vi "Perform Action.vi"(8 "error in":errorcluster, 10 "Input":variant, 11 "AI Voltage DAQmx Cont CFG Simulated in":refnum<class "AI Voltage DAQmx Cont CFG Simulated.lvclass">) -> (0 "error out":errorcluster, 2 "Output":variant, 3 "AI Voltage DAQmx Cont CFG Simulated out":refnum<class "AI Voltage DAQmx Cont CFG Simulated.lvclass">)   [LabVIEW 2023, in "DAQmx Simulated CFGs.lvlib" / "AI Voltage DAQmx Cont CFG Simulated.lvclass"]
uses:
  DAQmx/DAQmx BufferLastReadsDBL/DAQmx BufferLastReadsDBL.lvclass/DAQmx BufferLastReadsDBL.ctl
  DAQmx/DAQmx Base CFG/DAQmx Base CFG.lvclass/DAQmx Base CFG.ctl
  Configuration/Configuration Semaphore/CFG Semaphore.lvclass/CFG Semaphore.ctl
  <vilib>/JDP Science/JSONtext/Find Item.vi
  <vilib>/JDP Science/JSONtext/Next JSON Value.vi
  <vilib>/JDP Science/JSONtext/String Subset.vi
  <vilib>/JDP Science/JSONtext/Parsing/Advance past next JSON Value (inlined COPY).vi
  <vilib>/JDP Science/JSONtext/Parsing/Advance past whitespace.vi
  <vilib>/JDP Science/JSONtext/Parsing/Advance past String.vi
  <vilib>/JDP Science/JSONtext/Parsing/Advance past Number.vi
  <vilib>/JDP Science/JSONtext/Parsing/Advance past Line Ending.vi
  <vilib>/JDP Science/JSONtext/Parsing/Parse Full Path or Item Name.vi
  <vilib>/JDP Science/JSONtext/Parsing/Advance past Array.vi
  <vilib>/JDP Science/JSONtext/Parsing/Advance past Object.vi
  <vilib>/JDP Science/JSONtext/support/Error Cluster From Code.vi
  <vilib>/JDP Science/JSONtext/Offset/Find Item Locations by Path.vi
  <vilib>/JDP Science/JSONtext/JSON text to Variant.vi
  <vilib>/DAQmx/miscellaneous.llb/DAQmx Fill In Error Info.vi
  <vilib>/JDP Science/JSONtext/LVClass Serializer/JSONtext LVClass Serializer.lvclass
  AI Voltage DAQmx Cont CFG Simulated.lvclass
  AI Voltage DAQmx Cont CFG Simulated.lvclass/AI Voltage DAQmx Cont CFG Simulated.ctl
  45e9973d-d2d9-4ea1-97eb-1b57adbb2603.vi
  DAQmx/DAQmx BufferLastReadsDBL/DAQmx BufferLastReadsDBL.lvclass
  DAQmx/BufferLastReadingsDBL/BufferLastReadsDBL.lvclass
  Configuration/Configuration JSON/Configuration JSON Base/CFG JSON.lvclass
  0cc4d47a-a0da-4a28-b8ba-3adaf38567aa.vi
  D:/git/HAL/HAL GOOP4/AI/AI Voltage DAQmx Cont CFG/AI Voltage DAQmx Cont CFG.lvclass
  D:/git/HAL/HAL GOOP4/DAQmx/DAQmx BufferLastReadsDBL/DAQmx BufferLastReadsDBL.lvclass
  D:/git/HAL/HAL GOOP4/DAQmx/DAQmx Base CFG/DAQmx Base CFG.lvclass
  D:/git/HAL/HAL GOOP4/CFG Target/CFG Target.lvclass
  D:/git/HAL/HAL GOOP4/Configuration/Configuration Semaphore/CFG Semaphore.lvclass
  D:/git/HAL/HAL GOOP4/Configuration/Configuration JSON/Configuration JSON Base/CFG JSON.lvclass
  D:/git/HAL/HAL GOOP4/Interfaces/IConfigure/IConfigure.lvclass
  D:/git/HAL/HAL GOOP4/AI/AI Voltage DAQmx Cont CFG Simulated/AI Voltage DAQmx Cont CFG Simulated.lvclass
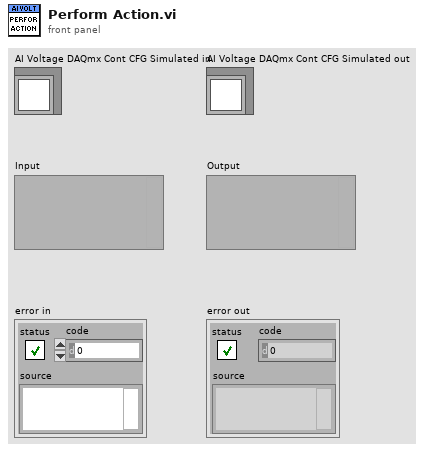
[diagram p1: front panel]
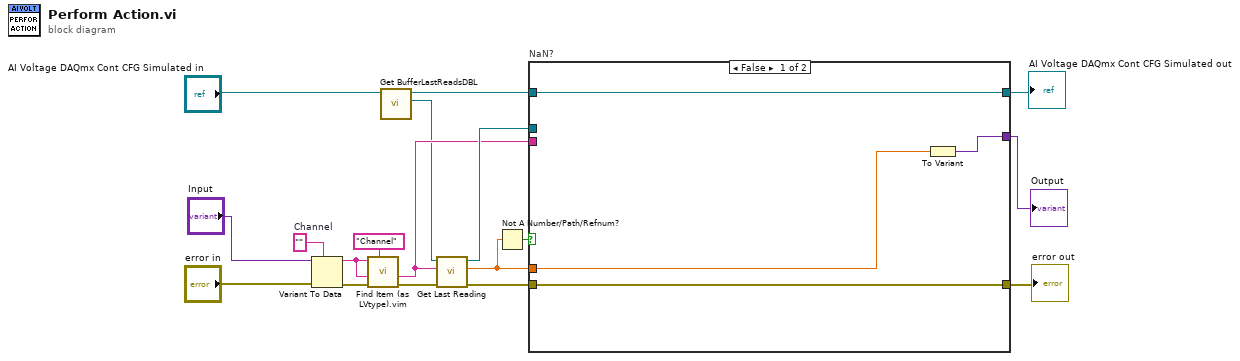
[diagram p0: block diagram]
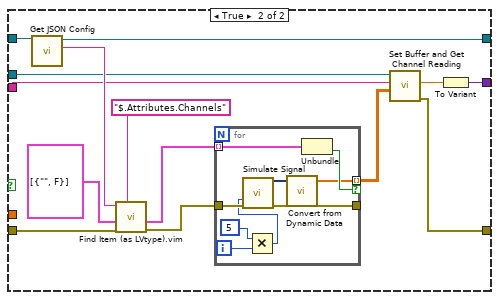
[diagram p2: hidden frame]
diagram:
  w14 = ""  # Channel
  n1 = Variant To Data(error in="error in", type=w14, Variant="Input") -> (data=w11:string, error out=w12:errorcluster)
  n2 = call "Find Item (as LVtype).vim"("$Path or Item Name"="Channel", "error in (no error)"=w12, "Data Type and Default Value"=w11, "JSON"=w11) -> ("error out"=w13:errorcluster, "Data"=w9:string)  [unwired: 4 in, 2 out]
  n3 = call "Get BufferLastReadsDBL.vi"("DAQmx BufferLastReadsDBL in"="AI Voltage DAQmx Cont CFG Simulated in") -> ("BufferLastReadsDBL.lvclass"=w7:refnum<class "BufferLastReadsDBL.lvclass">, "DAQmx BufferLastReadsDBL out"=w8:refnum<class "AI Voltage DAQmx Cont CFG Simulated.lvclass">)  [unwired: 9 in]
  n4 = call-dynamic "Get Last Reading.vi"("error in"=w13, "Channel"=w9, "BufferLastReadingsDBL in"=w7) -> ("error out"=w16:errorcluster, "Reading"=w17:dbl, "BufferLastReadingsDBL out"=w15:refnum<class "BufferLastReadsDBL.lvclass">)  [unwired: 6 in]
  n5 = Not A Number/Path/Refnum?(number/path/refnum=w17) -> (NaN/Path/Refnum?=w18:bool)
  n6 = case "NaN?" shown="False" w18 {
    tunnel: [w19 w36] -> w1
    tunnel: [w20 w30] -> w3
    tunnel: w8 -> [w20 w31]
    tunnel: w15 -> [_ w29]
    tunnel: [w21 w35] -> w2
    tunnel: w17 -> [w22 _]
    tunnel: w16 -> [w19 w27]
    tunnel: w9 -> [_ w23]
    frame False {
      n7 = To Variant(anything=w22) -> (Variant=w21:variant)
    }
    frame True {
      n8 = call "Get JSON Config.vi"("CFG Base in"=w31) -> ("<JSON>Config>"=w33:string, "CFG Base out"=w30:refnum<class "AI Voltage DAQmx Cont CFG Simulated.lvclass">)  [unwired: 9 in]
      n9 = call "Find Item (as LVtype).vim"("$Path or Item Name"="$.Attributes.Channels", "error in (no error)"=w27, "Data Type and Default Value"=cluster{"Name":string, "Enabled":bool}[] [{"Name"="", "Enabled"=FALSE}], "JSON"=w33) -> ("error out"=w26:errorcluster, "Data"=w25:cluster{"Name":string, "Enabled":bool}[])  [unwired: 4 in, 2 out]
      n10 = for {
        tunnel: w25 -> [w45] mode=indexing
        tunnel: w26 -> [w44]
        tunnel: [w43] -> _
        tunnel: [w38] -> w24 mode=indexing if=w42
        i -> [w41]
        n11 = Multiply(x=5, y=w41) -> (x*y=w37:i32)
        n12 = call "Simulate Signal"("Phase"=w37, "error in (no error)"=w44) -> ("Sine with Uniform Noise"=w39:dynamicdata, "error out"=w43:errorcluster)  [unwired: 12 in]
        n13 = call "Convert from Dynamic Data"("Dynamic Data Type"=w39) -> ("Array"=w38:dbl[])  [unwired: 3 in]
        n14 = Unbundle(w45) -> ("Enabled"=w42:bool)  [unwired: 1 out]
      }
      n15 = call-dynamic "Set Buffer and Get Channel Reading.vi"("Readings"=w24, "Channel Ident"=w23, "BufferLastReadingsDBL in"=w29) -> ("error out"=w36:errorcluster, "Reading"=w34:dbl)  [unwired: 6 in, 1 out]
      n16 = To Variant(anything=w34) -> (Variant=w35:variant)
    }
  }
  "error out" <- w1
  "AI Voltage DAQmx Cont CFG Simulated out" <- w3
  "Output" <- w2
